vi "CheckStringFormat.vi"(9 "Type":T1(ring), 10 "HighLimit":string, 11 "LowLimit":string) -> (3 "status":bool)   [LabVIEW 2019, in "TestSetup.lvlib" / "TestSetup.lvclass"]
uses:
  TestSetup.lvclass
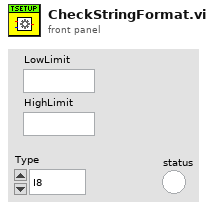
[diagram p1: front panel]
types:
  T1 = enum16{"I8", "I16", "I32", "I64", "U8", "U16", "U32", "U64", "Double Float", "Boolean", "String", "Numeric Array", "String Array"}
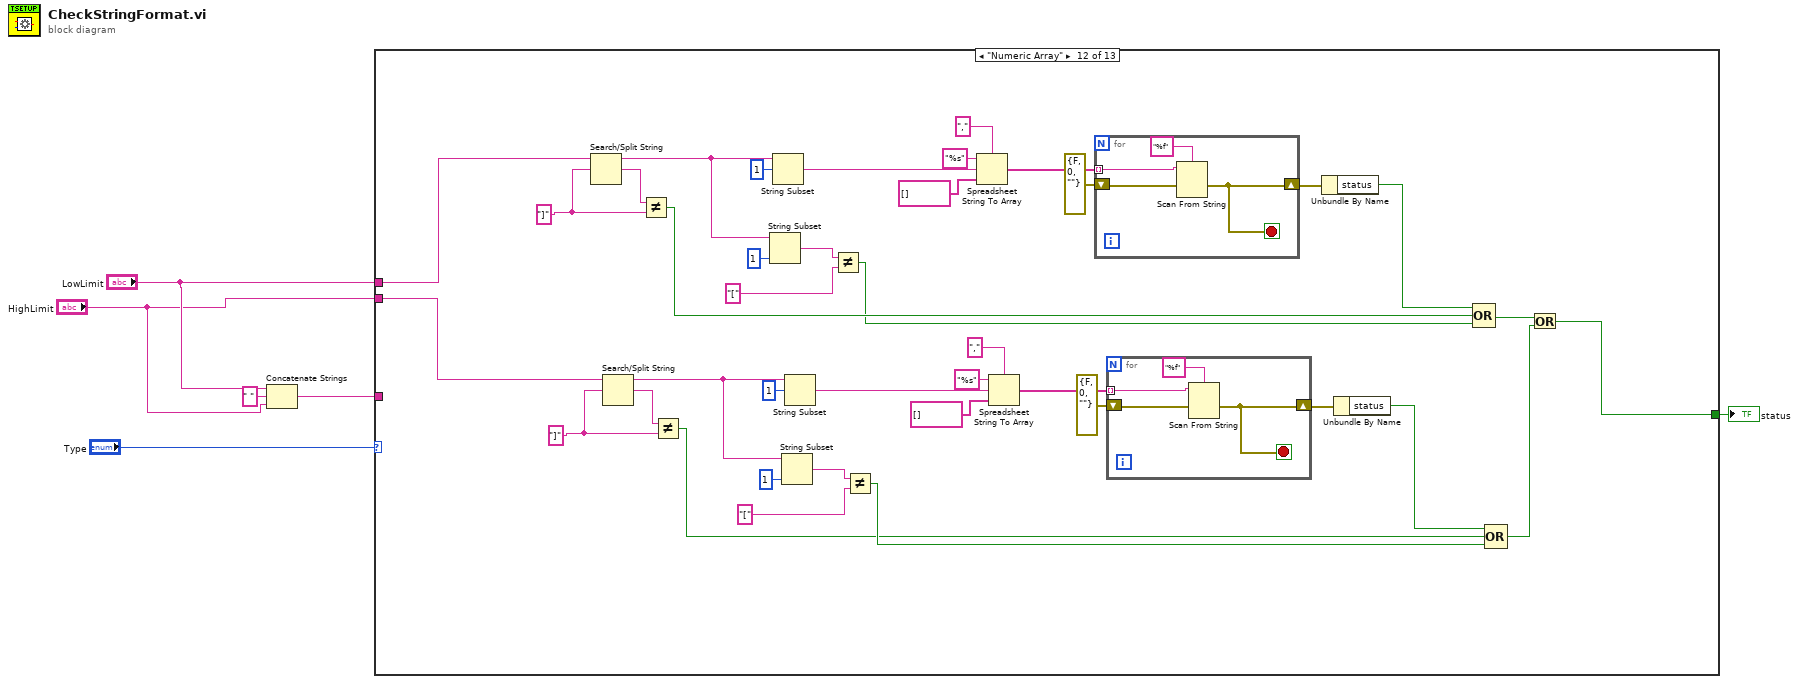
[diagram p0: block diagram]
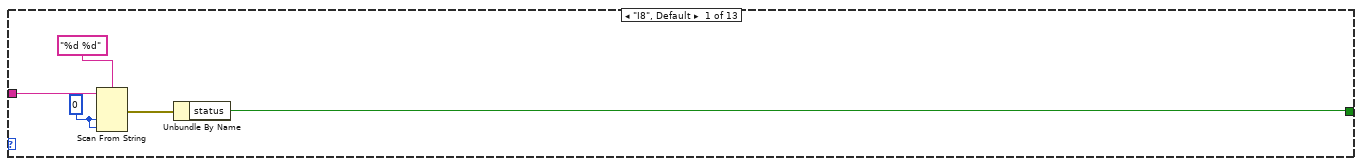
[diagram p2: hidden frame]
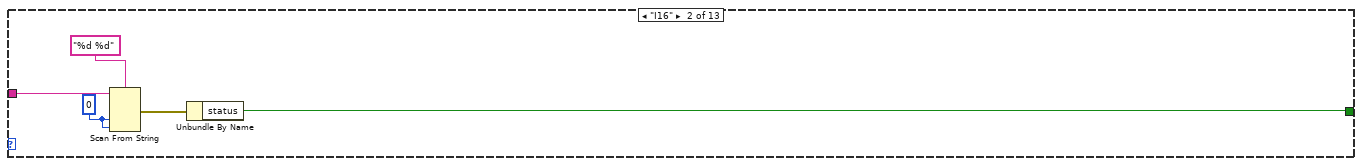
[diagram p3: hidden frame]
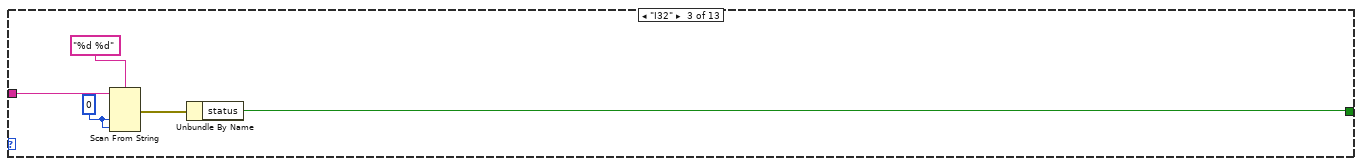
[diagram p4: hidden frame]
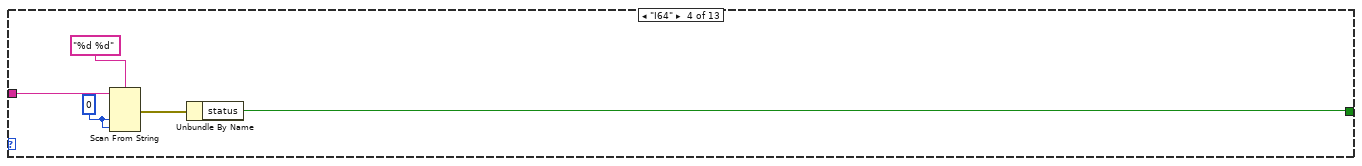
[diagram p5: hidden frame]
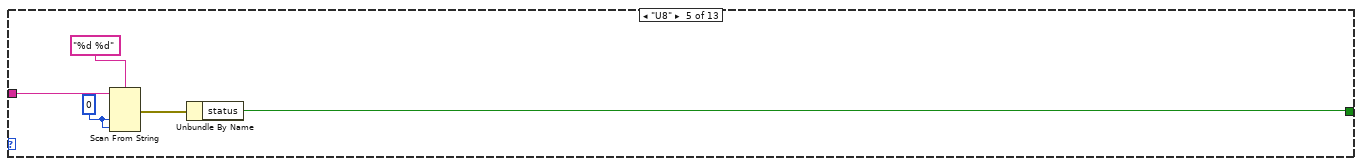
[diagram p6: hidden frame]
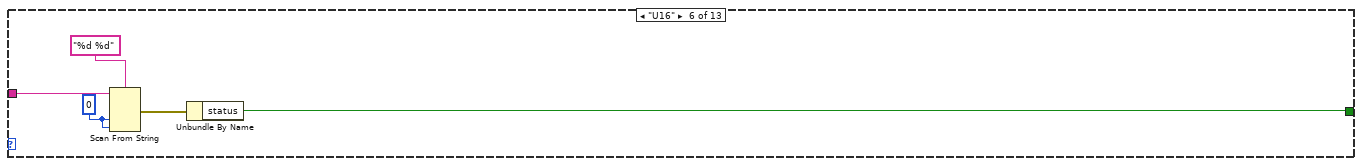
[diagram p7: hidden frame]
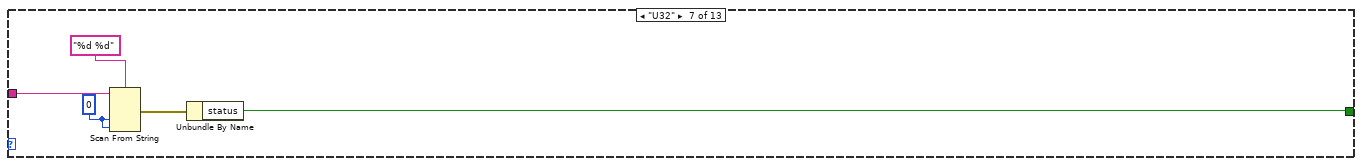
[diagram p8: hidden frame]
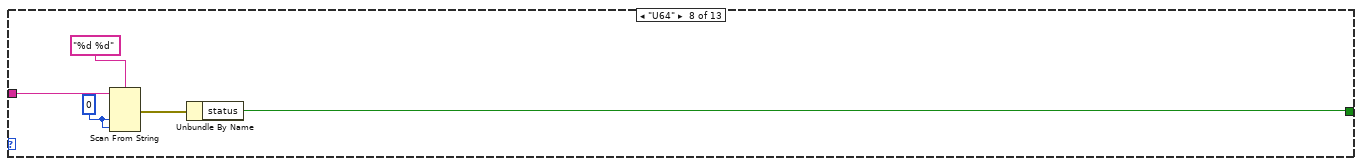
[diagram p9: hidden frame]
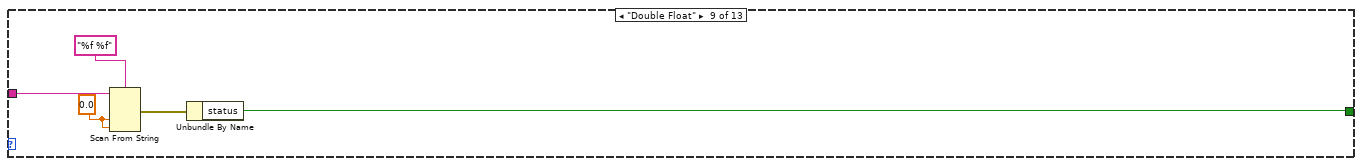
[diagram p10: hidden frame]
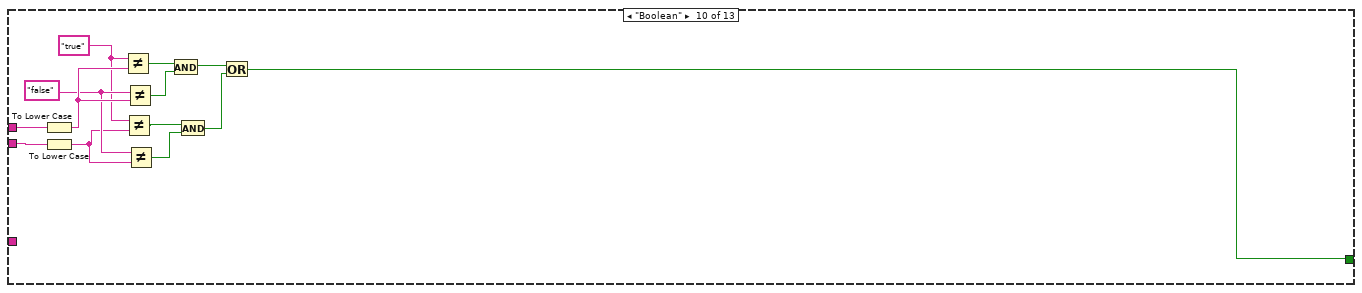
[diagram p11: hidden frame]
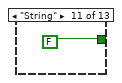
[diagram p12: hidden frame]
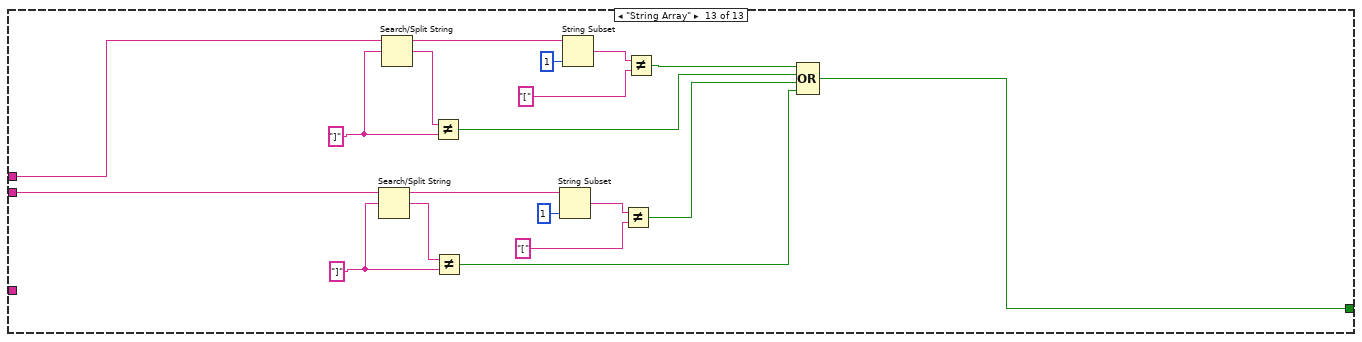
[diagram p13: hidden frame]
diagram:
  n1 = Concatenate Strings("LowLimit", " " ("string"), "HighLimit") -> (w5:string)
  n2 = case shown="\"Numeric Array\"" "Type" {
    tunnel: w5 -> [w9 w13 w18 w23 w28 w33 w38 w43 w48 _ _ _ _]
    tunnel: [w7 w12 w17 w22 w27 w32 w37 w42 w47 w52 FALSE w66 w113] -> w4
    tunnel: "HighLimit" -> [_ _ _ _ _ _ _ _ _ w61 _ w69 w118]
    tunnel: "LowLimit" -> [_ _ _ _ _ _ _ _ _ w60 _ w87 w125]
    frame "I8", Default {
      w10 = i8 0
      n3 = Scan From String(format string="%d %d", input string=w9, default 1=w10, default 2=w10) -> (error out=w8:errorcluster)  [unwired: 4 in, 2 out]
      n4 = Unbundle By Name(w8) -> ("status"=w7:bool)
    }
    frame "I16" {
      w15 = i16 0
      n5 = Scan From String(format string="%d %d", input string=w13, default 1=w15, default 2=w15) -> (error out=w14:errorcluster)  [unwired: 4 in, 2 out]
      n6 = Unbundle By Name(w14) -> ("status"=w12:bool)
    }
    frame "I32" {
      w20 = 0
      n7 = Scan From String(format string="%d %d", input string=w18, default 1=w20, default 2=w20) -> (error out=w19:errorcluster)  [unwired: 4 in, 2 out]
      n8 = Unbundle By Name(w19) -> ("status"=w17:bool)
    }
    frame "I64" {
      w25 = i64 0
      n9 = Scan From String(format string="%d %d", input string=w23, default 1=w25, default 2=w25) -> (error out=w24:errorcluster)  [unwired: 4 in, 2 out]
      n10 = Unbundle By Name(w24) -> ("status"=w22:bool)
    }
    frame "U8" {
      w30 = u8 0
      n11 = Scan From String(format string="%d %d", input string=w28, default 1=w30, default 2=w30) -> (error out=w29:errorcluster)  [unwired: 4 in, 2 out]
      n12 = Unbundle By Name(w29) -> ("status"=w27:bool)
    }
    frame "U16" {
      w35 = u16 0
      n13 = Scan From String(format string="%d %d", input string=w33, default 1=w35, default 2=w35) -> (error out=w34:errorcluster)  [unwired: 4 in, 2 out]
      n14 = Unbundle By Name(w34) -> ("status"=w32:bool)
    }
    frame "U32" {
      w40 = u32 0
      n15 = Scan From String(format string="%d %d", input string=w38, default 1=w40, default 2=w40) -> (error out=w39:errorcluster)  [unwired: 4 in, 2 out]
      n16 = Unbundle By Name(w39) -> ("status"=w37:bool)
    }
    frame "U64" {
      w45 = u64 0
      n17 = Scan From String(format string="%d %d", input string=w43, default 1=w45, default 2=w45) -> (error out=w44:errorcluster)  [unwired: 4 in, 2 out]
      n18 = Unbundle By Name(w44) -> ("status"=w42:bool)
    }
    frame "Double Float" {
      w50 = 0.0
      n19 = Scan From String(format string="%f %f", input string=w48, default 1=w50, default 2=w50) -> (error out=w49:errorcluster)  [unwired: 4 in, 2 out]
      n20 = Unbundle By Name(w49) -> ("status"=w47:bool)
    }
    frame "Boolean" {
      w63 = "false"
      w62 = "true"
      n21 = To Lower Case(string=w60) -> (all lower case string=w64:string)
      n22 = To Lower Case(string=w61) -> (all lower case string=w59:string)
      n23 = Not Equal?(x=w62, y=w64) -> (x != y?=w58:bool)
      n24 = Not Equal?(x=w62, y=w59) -> (x != y?=w56:bool)
      n25 = Not Equal?(x=w63, y=w64) -> (x != y?=w57:bool)
      n26 = Not Equal?(x=w63, y=w59) -> (x != y?=w55:bool)
      n27 = And(x=w58, y=w57) -> (x .and. y?=w54:bool)
      n28 = And(x=w56, y=w55) -> (x .and. y?=w53:bool)
      n29 = Or(x=w54, y=w53) -> (x .or. y?=w52:bool)
    }
    frame "String" {
    }
    frame "Numeric Array" {
      w76 = "]" ("regular expression")
      w98 = "]" ("regular expression")
      n30 = Search/Split String(string=w87, search string/char (-)=w98) -> (substring before match=w103:string, match + rest of string=w99:string)  [unwired: 1 in, 1 out]
      n31 = Search/Split String(string=w69, search string/char (-)=w76) -> (substring before match=w71:string, match + rest of string=w75:string)  [unwired: 1 in, 1 out]
      n32 = Not Equal?(x=w99, y=w98) -> (x != y?=w89:bool)
      n33 = Not Equal?(x=w75, y=w76) -> (x != y?=w85:bool)
      n34 = String Subset(string=w103, length (rest)=1 ("length (rest)")) -> (substring=w101:string)  [unwired: 1 in]
      n35 = String Subset(string=w103, offset (0)=1) -> (substring=w97:string)  [unwired: 1 in]
      n36 = String Subset(string=w71, length (rest)=1 ("length (rest)")) -> (substring=w73:string)  [unwired: 1 in]
      n37 = String Subset(string=w71, offset (0)=1) -> (substring=w77:string)  [unwired: 1 in]
      n38 = Not Equal?(x=w101, y="[" ("regular expression")) -> (x != y?=w88:bool)
      n39 = Not Equal?(x=w73, y="[" ("regular expression")) -> (x != y?=w86:bool)
      n40 = Spreadsheet String To Array(delimiter (Tab)=",", format string="%s", spreadsheet string=w97, array type (2D Dbl)=string[] []) -> (array=w93:string[])
      n41 = Spreadsheet String To Array(delimiter (Tab)=",", format string="%s", spreadsheet string=w77, array type (2D Dbl)=string[] []) -> (array=w81:string[])
      n42 = for {
        tunnel: w93 -> [w112] mode=indexing
        shift-right: [w109] -> w91
        shift-left: errorcluster {"status"=FALSE, "code"=0, "source"=""} ("error IO") -> [w110]
        stop <- w109 stop-if-true
        n43 = Scan From String(format string="%f", input string=w112, error in=w110) -> (error out=w109:errorcluster)  [unwired: 3 in, 2 out]
      }
      n44 = for {
        tunnel: w81 -> [w108] mode=indexing
        shift-right: [w105] -> w83
        shift-left: errorcluster {"status"=FALSE, "code"=0, "source"=""} ("error IO") -> [w106]
        stop <- w105 stop-if-true
        n45 = Scan From String(format string="%f", input string=w108, error in=w106) -> (error out=w105:errorcluster)  [unwired: 3 in, 2 out]
      }
      n46 = Unbundle By Name(w91) -> ("status"=w90:bool)
      n47 = Unbundle By Name(w83) -> ("status"=w84:bool)
      n48 = Compound Arithmetic op=OR(w90, w89, w88) -> (w68:bool)
      n49 = Compound Arithmetic op=OR(w84, w85, w86) -> (w67:bool)
      n50 = Or(x=w68, y=w67) -> (x .or. y?=w66:bool)
    }
    frame "String Array" {
      w124 = "]" ("regular expression")
      w126 = "]" ("regular expression")
      n51 = Search/Split String(string=w118, search string/char (-)=w124) -> (substring before match=w119:string, match + rest of string=w123:string)  [unwired: 1 in, 1 out]
      n52 = Search/Split String(string=w125, search string/char (-)=w126) -> (substring before match=w131:string, match + rest of string=w127:string)  [unwired: 1 in, 1 out]
      n53 = Not Equal?(x=w127, y=w126) -> (x != y?=w116:bool)
      n54 = Not Equal?(x=w123, y=w124) -> (x != y?=w114:bool)
      n55 = String Subset(string=w119, length (rest)=1 ("length (rest)")) -> (substring=w121:string)  [unwired: 1 in]
      n56 = String Subset(string=w131, length (rest)=1 ("length (rest)")) -> (substring=w129:string)  [unwired: 1 in]
      n57 = Not Equal?(x=w121, y="[" ("regular expression")) -> (x != y?=w115:bool)
      n58 = Not Equal?(x=w129, y="[" ("regular expression")) -> (x != y?=w117:bool)
      n59 = Compound Arithmetic op=OR(w117, w116, w115, w114) -> (w113:bool)
    }
  }
  "status" <- w4
